vi "Autonomous Independent.vi"() -> ()   [LabVIEW 2015]
doc: "This VI is called when autonomous begins, and will automatically be terminated when autonomous ends. You can carry out timed or sensor driven robot movement independently without needing to return to the caller."
uses:
  <vilib>/Rock Robotics/WPI/Utilities/WPI_GetSetVariantRefNum.vi
  <vilib>/Rock Robotics/Network Tables/NT Write Numeric Array.vi
  <vilib>/Rock Robotics/Network Tables/NT Read String.vi
panel:
  in  "Enum 2":T1(ring)
  in  "Enum":T2(ring)
  # "Be sure to right-click and choose Data Operations>>Make Current Value default if you want to save the array values with the VI"
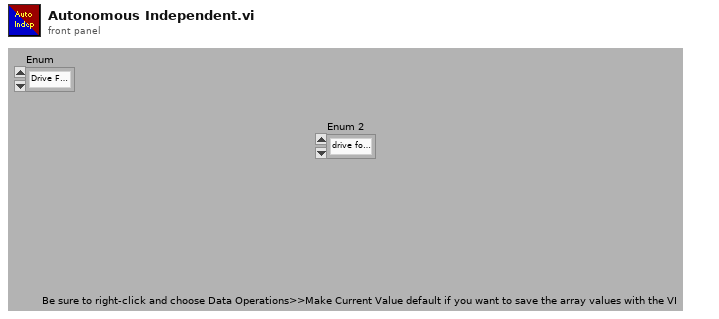
[diagram p1: front panel]
types:
  T1 = enum16{"drive forward", "extend elevator", "drive forward and hook DB", "drive backward and go down", "drive forward some"}
  T2 = enum16{"Drive Forward", "Hook Door", "Drive Backward", "Spin Longway or Something", "Drive Backwards"}
  T3 = typedef "WPI_RobotDriveDevRef.ctl" = cluster{"DevStatus":errorcluster, "Motors[]":T4[], "Square Inputs":bool, "Max Output":dbl}
  T4 = typedef "WPI_MotorControlDeviceRef.ctl" = cluster{"DeviceStatus":errorcluster, "Type":T5, "PWM":cluster{"PWM Channel":T6, "DeadBand":T7}, "CAN":cluster{"Device Number":u8, "Control Mode":T8, "Semaphore":T9, "Max Vout":dbl, "TalonSRX Control Mode":T10}, "Invert":bool}
  T5 = typedef "WPI_MotorControlType.ctl" = enum16{"PWM", "CAN", "CANTalonSRX"}
  T6 = typedef "FPGA_DIOPWMChannel.ctl" = enum8{"PWM 0", "PWM 1", "PWM 2", "PWM 3", "PWM 4", "PWM 5", "PWM 6", "PWM 7", "PWM 8", "PWM 9", "PWM MXP 0", "PWM MXP 1", "PWM MXP 2", "PWM MXP 3", "PWM MXP 4", "PWM MXP 5", "PWM MXP 6", "PWM MXP 7", "PWM MXP 8", "PWM MXP 9", "Invalid"}
  T7 = typedef "WPI_PWMDeadband.ctl" = cluster{"Name":string, "maxPositivePwm":i32, "minPositivePwm":i32, "centerPwm":i32, "maxNegativePwm":i32, "minNegativePwm":i32, "angularRange":u16}
  T8 = typedef "WPI_CANJaguar_ControlMode.ctl" = enum8{"Percent VBus", "Current", "Speed", "Position", "Voltage"}
  T9 = typedef "Semaphore RefNum" = refnum<k1>
  T10 = typedef "WPI_CANTalonSRX_APIControlMode.ctl" = enum8{"Percent VBus", "Speed", "Position", "Slave", "Unchanged / Invalid", "Voltage Compensation", "Current", "Motion Profile"}
  T11 = typedef "WPI_EncoderDevRef.ctl" = cluster{"DevStatus":errorcluster, "EncoderIndex":T12, "CounterIndex":T13, "DistancePerCount":dbl, "Decoding Type":T14}
  T12 = typedef "FPGA_EncoderIdx.ctl" = enum8{"Enc 0", "Enc 1", "Enc 2", "Enc 3", "Enc 4", "Enc 5", "Enc 6", "Enc 7", "Invalid"}
  T13 = typedef "FPGA_CounterCtrSystemIndex.ctl" = enum8{"Ctr 0", "Ctr 1", "Ctr 2", "Ctr 3", "Ctr 4", "Ctr 5", "Ctr 6", "Ctr 7", "Invalid"}
  T14 = typedef "WPI_EncoderType.ctl" = enum16{"1x", "2x", "4x"}
  T15 = typedef "WPI_JoystickDevRef.ctl" = cluster{"Device":T16}
  T16 = typedef "WPI_JoystickDeviceEnum.ctl" = enum16{"USB 0", "USB 1", "USB 2", "USB 3", "USB 4", "USB 5"}
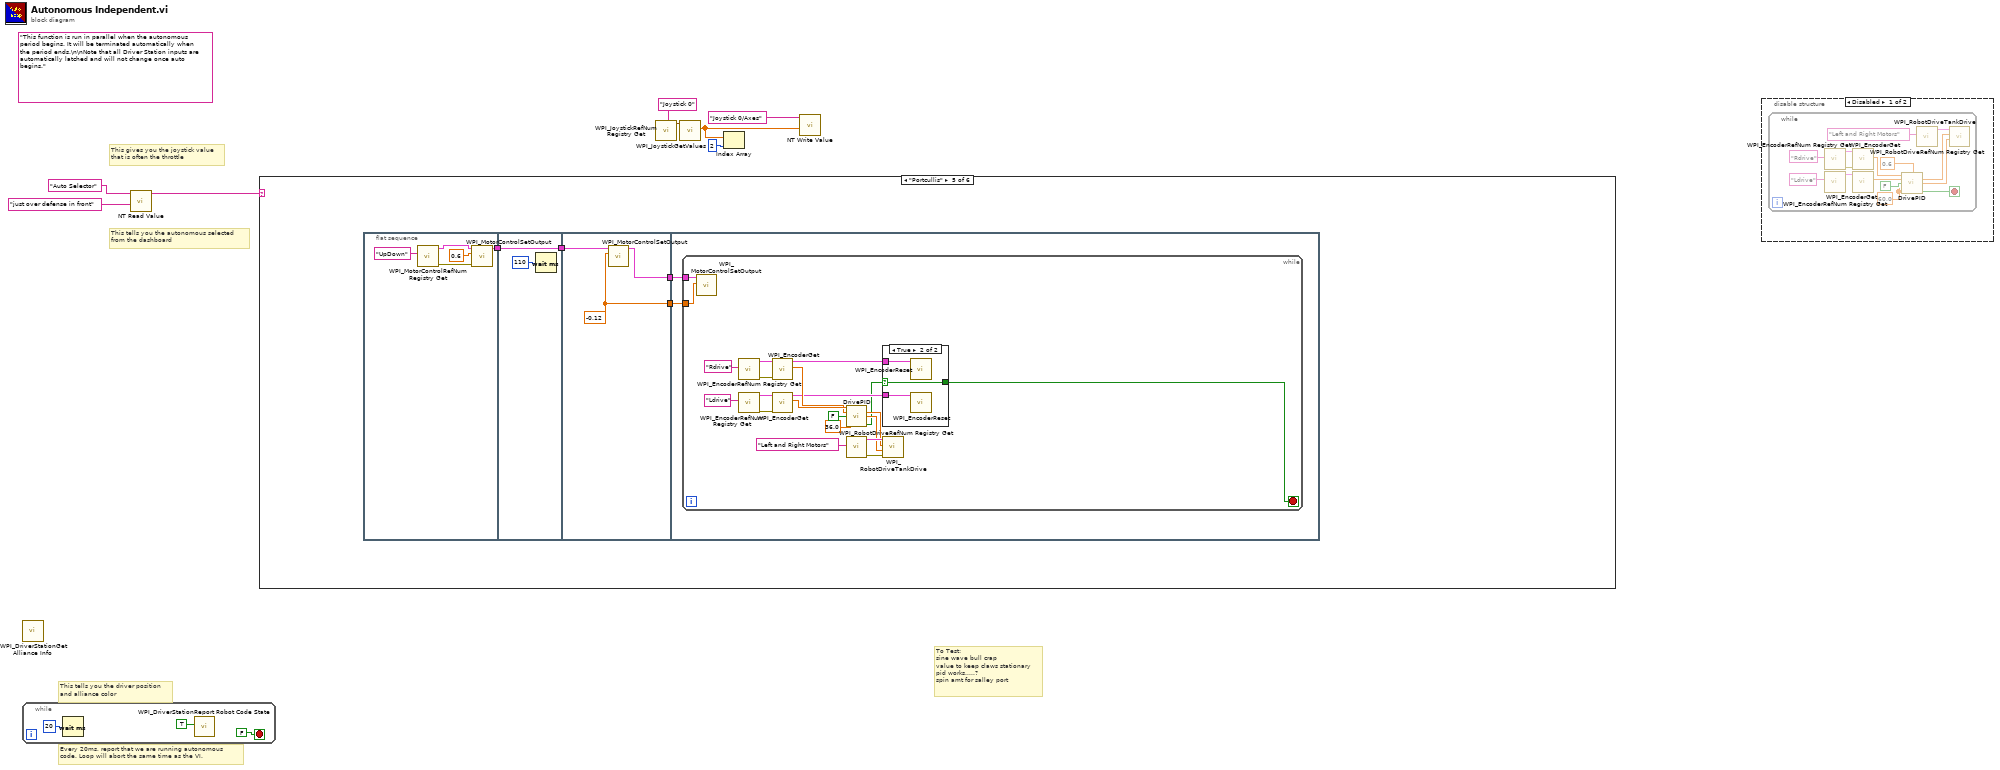
[diagram p0: block diagram]
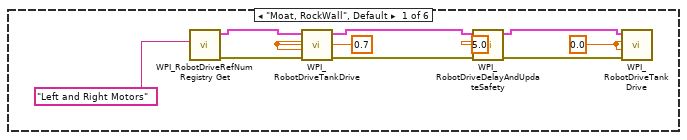
[diagram p2: hidden frame]
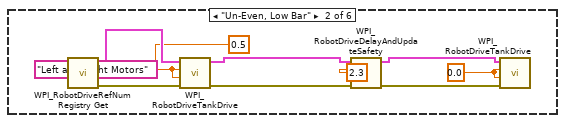
[diagram p3: hidden frame]
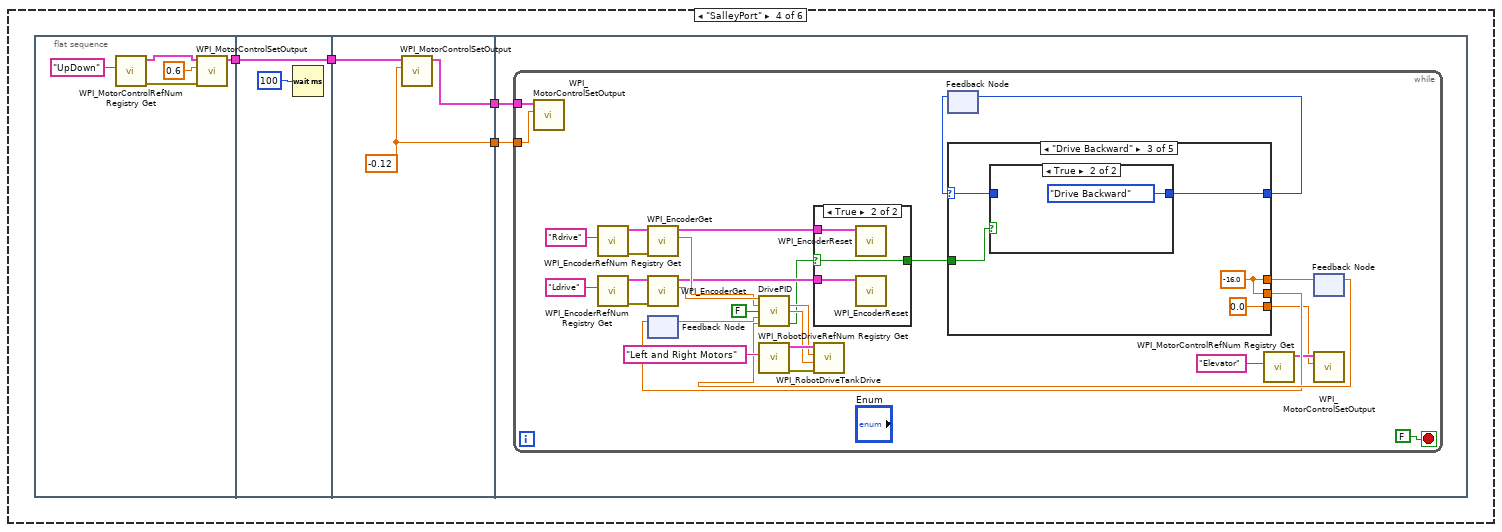
[diagram p5: hidden frame]
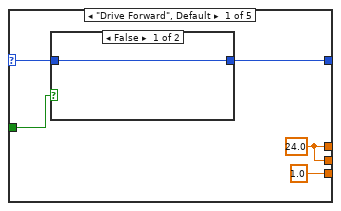
[diagram p6: hidden frame]
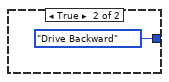
[diagram p7: hidden frame]
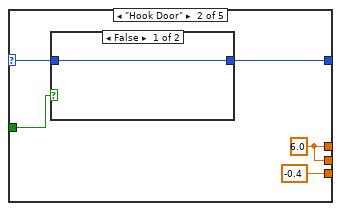
[diagram p8: hidden frame]
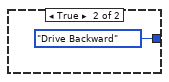
[diagram p9: hidden frame]
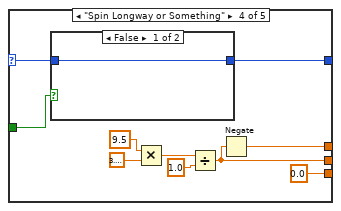
[diagram p11: hidden frame]
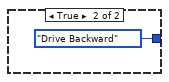
[diagram p12: hidden frame]
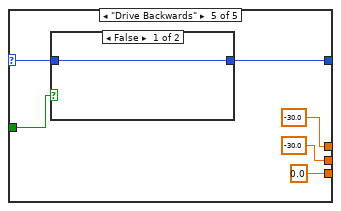
[diagram p13: hidden frame]
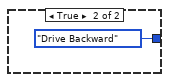
[diagram p14: hidden frame]
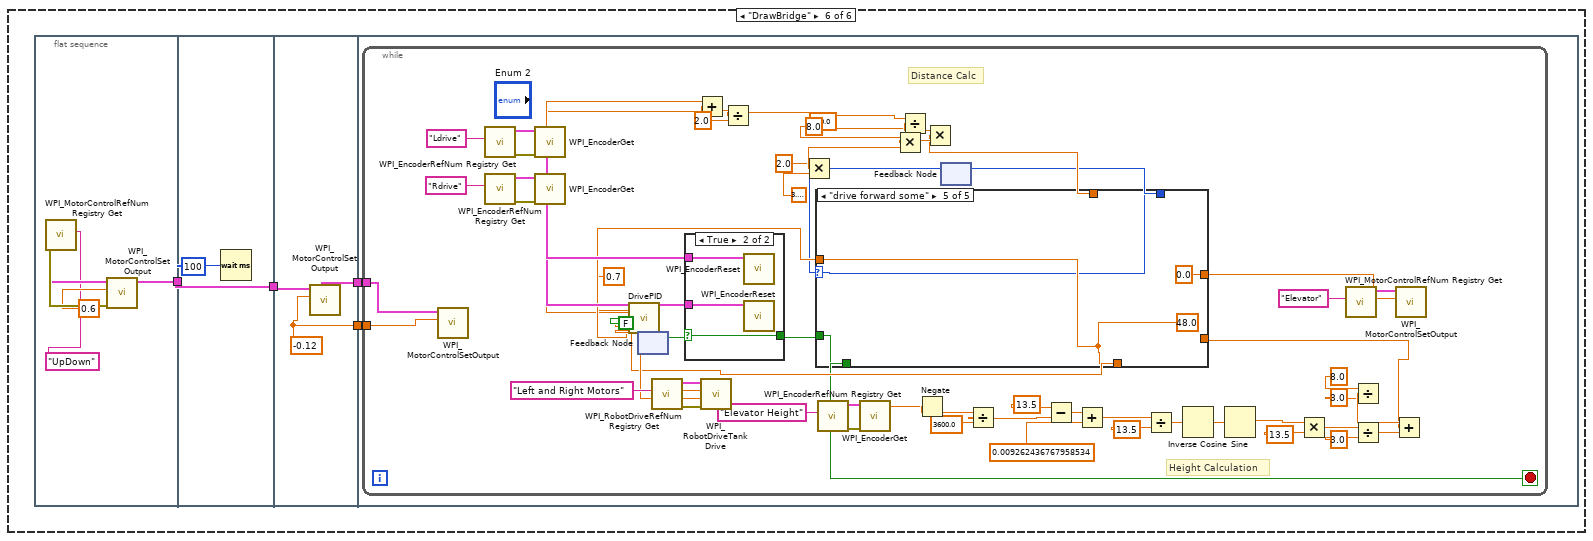
[diagram p17: hidden frame]
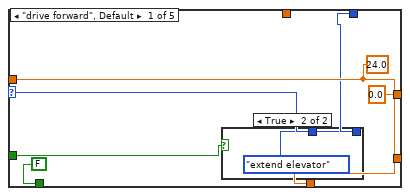
[diagram p19: hidden frame]
diagram:
  (unwired) "This function is run in parallel when the autonomous period begins. It will be terminated automatically when the period ends.\n\nNote that all Driver Station inputs are automatically latched and will not change once auto begins."
  # "To Test:\nsine wave bull crap\nvalue to keep claws stationary\npid works.....?\nspin amt for salley port"
  # "This tells you the autonomous selected\nfrom the dashboard"
  # "Every 20ms, report that we are running autonomous\ncode. Loop will abort the same time as the VI."
  # "This gives you the joystick value\nthat is often the throttle"
  # "This tells you the driver position\nand alliance color"
  n1 = while {
    stop <- FALSE stop-if-true
    n2 = Wait (ms)(milliseconds to wait=u32 20) -> ()  [unwired: 1 out]
    n3 = call <vilib>:"WPI_DriverStationReport Robot Code State.vi"("Autonomous"=TRUE) -> ()  [unwired: 10 in, 1 out]
  }
  n4 = call <vilib>:"WPI_DriverStationGet Alliance Info.vi"() -> ()  [unwired: 12 out]
  n5 = call-poly <vilib>:"NT Read Value.vi"("Default Value"="just over defense in front", "Name"="Auto Selector") -> ("String"=w1:string)  [unwired: 8 in, 1 out]
  n6 = case shown="\"Portcullis\"" w1 {
    frame "Moat, RockWall", Default {
      w15 = 0.0 ("Left axis value")
      w16 = 0.7 ("Left axis value")
      n7 = call <vilib>:"WPI_RobotDriveRefNum Registry Get.vi"("refnum name"="Left and Right Motors") -> ("error out"=w18:errorcluster, "RobotDriveDevRef"=w21:T3)  [unwired: 9 in]
      n8 = call <vilib>:"WPI_RobotDriveTankDrive.vi"("error in (no error)"=w18, "Right axis value"=w16, "Left axis value"=w16, "RobotDriveDevRef"=w21) -> ("error out"=w17:errorcluster, "RobotDriveDevRef"=w19:T3)  [unwired: 5 in, 1 out]
      n9 = call <vilib>:"WPI_RobotDriveDelayAndUpdateSafety.vi"("error in (no error)"=w17, "Delay (s)"=5.0, "RobotDriveDevRef"=w19) -> ("error out"=w13:errorcluster, "RobotDriveDevRef 2"=w14:T3)  [unwired: 7 in]
      n10 = call <vilib>:"WPI_RobotDriveTankDrive.vi"("error in (no error)"=w13, "Right axis value"=w15, "Left axis value"=w15, "RobotDriveDevRef"=w14) -> ()  [unwired: 5 in, 3 out]
    }
    frame "Un-Even, Low Bar" {
      w22 = 0.5 ("Left axis value")
      w28 = 0.0 ("Left axis value")
      n11 = call <vilib>:"WPI_RobotDriveRefNum Registry Get.vi"("refnum name"="Left and Right Motors") -> ("error out"=w26:errorcluster, "RobotDriveDevRef"=w23:T3)  [unwired: 9 in]
      n12 = call <vilib>:"WPI_RobotDriveTankDrive.vi"("error in (no error)"=w26, "Right axis value"=w22, "Left axis value"=w22, "RobotDriveDevRef"=w23) -> ("error out"=w27:errorcluster, "RobotDriveDevRef"=w25:T3)  [unwired: 5 in, 1 out]
      n13 = call <vilib>:"WPI_RobotDriveDelayAndUpdateSafety.vi"("error in (no error)"=w27, "Delay (s)"=2.3, "RobotDriveDevRef"=w25) -> ("error out"=w30:errorcluster, "RobotDriveDevRef 2"=w29:T3)  [unwired: 7 in]
      n14 = call <vilib>:"WPI_RobotDriveTankDrive.vi"("error in (no error)"=w30, "Right axis value"=w28, "Left axis value"=w28, "RobotDriveDevRef"=w29) -> ()  [unwired: 5 in, 3 out]
    }
    frame "Toaster" {
    }
    frame "SalleyPort" {
      n15 = flat-sequence {
        tunnel: [w37] -> w35
        tunnel: w35 -> [w41]
        tunnel: [w41] -> w34
        tunnel: w34 -> [w45]
        tunnel: [w44] -> w33
        tunnel: [w43] -> w32
        tunnel: w33 -> [w47]
        tunnel: w32 -> [w46]
        frame #0 {
          n16 = call <vilib>:"WPI_MotorControlRefNum Registry Get.vi"("refnum name"="UpDown") -> ("error out"=w40:errorcluster, "MotorControlDevRef"=w39:T4)  [unwired: 9 in]
          n17 = call <vilib>:"WPI_MotorControlSetOutput.vi"("error in (no error)"=w40, "Output"=0.6, "MotorControlDevRef"=w39) -> ("MotorControlDevRef"=w37:T4)  [unwired: 6 in, 2 out]
        }
        frame #1 {
          n18 = Wait (ms)(milliseconds to wait=u32 100) -> ()  [unwired: 1 out]
        }
        frame #2 {
          w43 = -0.12 ("Output")
          n19 = call <vilib>:"WPI_MotorControlSetOutput.vi"("Output"=w43, "MotorControlDevRef"=w45) -> ("MotorControlDevRef"=w44:T4)  [unwired: 7 in, 2 out]
        }
        frame #3 {
          n20 = while {
            tunnel: w47 -> [w49]
            tunnel: w46 -> [w48]
            stop <- FALSE stop-if-true
            n21 = call <vilib>:"WPI_MotorControlSetOutput.vi"("Output"=w48, "MotorControlDevRef"=w49) -> ()  [unwired: 7 in, 3 out]
            n22 = call <vilib>:"WPI_EncoderRefNum Registry Get.vi"("refnum name"="Rdrive") -> ("error out"=w74:errorcluster, "EncoderDevRef"=w73:T11)  [unwired: 9 in]
            n23 = call <vilib>:"WPI_EncoderRefNum Registry Get.vi"("refnum name"="Ldrive") -> ("error out"=w76:errorcluster, "EncoderDevRef"=w75:T11)  [unwired: 9 in]
            n24 = call <vilib>:"WPI_EncoderGet.vi"("error in (no error)"=w74, "EncoderDevRef"=w73) -> ("Distance"=w69:dbl, "EncoderDevRef"=w62:T11)  [unwired: 4 in, 4 out]
            n25 = call <vilib>:"WPI_EncoderGet.vi"("error in (no error)"=w76, "EncoderDevRef"=w75) -> ("Distance"=w70:dbl, "EncoderDevRef"=w63:T11)  [unwired: 4 in, 4 out]
            n26 = feedback #1() -> (w56:dbl)  [unwired: 1 in]
            n27 = call <vilib>:"WPI_RobotDriveRefNum Registry Get.vi"("refnum name"="Left and Right Motors") -> ("error out"=w67:errorcluster, "RobotDriveDevRef"=w66:T3)  [unwired: 9 in]
            n28 = feedback #2() -> (w54:T2)  [unwired: 1 in]
            n29 = call <vilib>:"WPI_MotorControlRefNum Registry Get.vi"("refnum name"="Elevator") -> ("MotorControlDevRef"=w52:T4)  [unwired: 9 in, 1 out]
            n30 = feedback #3() -> (w60:dbl)  [unwired: 1 in]
            n31 = call "DrivePID.vi"("Ldrive Encoder"=w70, "Rdrive Encoder"=w69, "Compensate"=FALSE, "SetpointLeft"=w56, "SetpointRight"=w60) -> ("Left Out"=w65:dbl, "Right Out"=w64:dbl, "Done"=w59:bool)  [unwired: 8 in]
            n32 = case shown="True" w59 {
              selector: w59 -> [w119 w120]
              tunnel: w63 -> [_ w122]
              tunnel: w62 -> [_ w121]
              tunnel: [w119 w120] -> w58
              frame False {
              }
              frame True {
                n33 = call <vilib>:"WPI_EncoderReset.vi"("EncoderDevRef"=w121) -> ()  [unwired: 9 in, 2 out]
                n34 = call <vilib>:"WPI_EncoderReset.vi"("EncoderDevRef"=w122) -> ()  [unwired: 9 in, 2 out]
              }
            }
            n35 = call <vilib>:"WPI_RobotDriveTankDrive.vi"("error in (no error)"=w67, "Right axis value"=w64, "Left axis value"=w65, "RobotDriveDevRef"=w66) -> ()  [unwired: 5 in, 3 out]
            n36 = case shown="\"Drive Backward\"" w54 {
              selector: w54 -> [w81 w88 w95 w107 w115]
              tunnel: [w82 w89 w96 w108 w116] -> w55
              tunnel: w58 -> [w78 w87 w94 w106 w114]
              tunnel: [w80 w85 w92 w100 -30.0] -> w61
              tunnel: [w80 w85 w92 w101 -30.0] -> w57
              tunnel: [1.0 -0.4 0.0 0.0 0.0] -> w51
              frame "Drive Forward", Default {
                w80 = 24.0
                n37 = case shown="False" w78 {
                  tunnel: [w83 T2."Drive Backward" ("Enum")] -> w82
                  tunnel: w81 -> [w83 _]
                  frame False {
                  }
                  frame True {
                  }
                }
              }
              frame "Hook Door" {
                w85 = 6.0
                n38 = case shown="False" w87 {
                  tunnel: [w90 T2."Drive Backward" ("Enum")] -> w89
                  tunnel: w88 -> [w90 _]
                  frame False {
                  }
                  frame True {
                  }
                }
              }
              frame "Drive Backward" {
                w92 = -16.0
                n39 = case shown="True" w94 {
                  tunnel: [w97 T2."Drive Backward" ("Enum")] -> w96
                  tunnel: w95 -> [w97 _]
                  frame False {
                  }
                  frame True {
                  }
                }
              }
              frame "Spin Longway or Something" {
                n40 = case shown="False" w106 {
                  tunnel: [w109 T2."Drive Backward" ("Enum")] -> w108
                  tunnel: w107 -> [w109 _]
                  frame False {
                  }
                  frame True {
                  }
                }
                n41 = Multiply(x=9.5, y=3.141592653589793) -> (x*y=w104:dbl)
                n42 = Divide(x=w104, y=1.0) -> (x/y=w101:dbl)
                n43 = Negate(x=w101) -> (-x=w100:dbl)
              }
              frame "Drive Backwards" {
                n44 = case shown="False" w114 {
                  tunnel: [w117 T2."Drive Backward" ("Enum")] -> w116
                  tunnel: w115 -> [w117 _]
                  frame False {
                  }
                  frame True {
                  }
                }
              }
            }
            n45 = feedback-in #1(w57) -> ()
            n46 = feedback-in #2(w55) -> ()
            n47 = feedback-in #3(w61) -> ()
            n48 = call <vilib>:"WPI_MotorControlSetOutput.vi"("Output"=w51, "MotorControlDevRef"=w52) -> ()  [unwired: 7 in, 3 out]
          }
        }
      }
    }
    frame "Portcullis" {
      n49 = flat-sequence {
        tunnel: [w128] -> w126
        tunnel: w126 -> [w132]
        tunnel: [w132] -> w125
        tunnel: w125 -> [w136]
        tunnel: [w135] -> w124
        tunnel: [w134] -> w123
        tunnel: w124 -> [w138]
        tunnel: w123 -> [w137]
        frame #0 {
          n50 = call <vilib>:"WPI_MotorControlRefNum Registry Get.vi"("refnum name"="UpDown") -> ("error out"=w131:errorcluster, "MotorControlDevRef"=w130:T4)  [unwired: 9 in]
          n51 = call <vilib>:"WPI_MotorControlSetOutput.vi"("error in (no error)"=w131, "Output"=0.6, "MotorControlDevRef"=w130) -> ("MotorControlDevRef"=w128:T4)  [unwired: 6 in, 2 out]
        }
        frame #1 {
          n52 = Wait (ms)(milliseconds to wait=u32 110) -> ()  [unwired: 1 out]
        }
        frame #2 {
          w134 = -0.12 ("Output")
          n53 = call <vilib>:"WPI_MotorControlSetOutput.vi"("Output"=w134, "MotorControlDevRef"=w136) -> ("MotorControlDevRef"=w135:T4)  [unwired: 7 in, 2 out]
        }
        frame #3 {
          n54 = while {
            tunnel: w138 -> [w142]
            tunnel: w137 -> [w141]
            stop <- w140 stop-if-true
            w139 = 36.0 ("SetpointLeft")
            n55 = call <vilib>:"WPI_MotorControlSetOutput.vi"("Output"=w141, "MotorControlDevRef"=w142) -> ()  [unwired: 7 in, 3 out]
            n56 = call <vilib>:"WPI_EncoderRefNum Registry Get.vi"("refnum name"="Rdrive") -> ("error out"=w156:errorcluster, "EncoderDevRef"=w155:T11)  [unwired: 9 in]
            n57 = call <vilib>:"WPI_EncoderRefNum Registry Get.vi"("refnum name"="Ldrive") -> ("error out"=w158:errorcluster, "EncoderDevRef"=w157:T11)  [unwired: 9 in]
            n58 = call <vilib>:"WPI_EncoderGet.vi"("error in (no error)"=w156, "EncoderDevRef"=w155) -> ("Distance"=w151:dbl, "EncoderDevRef"=w144:T11)  [unwired: 4 in, 4 out]
            n59 = call <vilib>:"WPI_EncoderGet.vi"("error in (no error)"=w158, "EncoderDevRef"=w157) -> ("Distance"=w152:dbl, "EncoderDevRef"=w145:T11)  [unwired: 4 in, 4 out]
            n60 = call "DrivePID.vi"("Ldrive Encoder"=w152, "Rdrive Encoder"=w151, "Compensate"=FALSE, "SetpointLeft"=w139, "SetpointRight"=w139) -> ("Left Out"=w147:dbl, "Right Out"=w146:dbl, "Done"=w143:bool)  [unwired: 8 in]
            n61 = call <vilib>:"WPI_RobotDriveRefNum Registry Get.vi"("refnum name"="Left and Right Motors") -> ("error out"=w149:errorcluster, "RobotDriveDevRef"=w148:T3)  [unwired: 9 in]
            n62 = case shown="True" w143 {
              selector: w143 -> [w160 w161]
              tunnel: w145 -> [_ w163]
              tunnel: w144 -> [_ w162]
              tunnel: [w160 w161] -> w140
              frame False {
              }
              frame True {
                n63 = call <vilib>:"WPI_EncoderReset.vi"("EncoderDevRef"=w162) -> ()  [unwired: 9 in, 2 out]
                n64 = call <vilib>:"WPI_EncoderReset.vi"("EncoderDevRef"=w163) -> ()  [unwired: 9 in, 2 out]
              }
            }
            n65 = call <vilib>:"WPI_RobotDriveTankDrive.vi"("error in (no error)"=w149, "Right axis value"=w146, "Left axis value"=w147, "RobotDriveDevRef"=w148) -> ()  [unwired: 5 in, 3 out]
          }
        }
      }
    }
    frame "DrawBridge" {
      n66 = flat-sequence {
        tunnel: [w169] -> w167
        tunnel: w167 -> [w173]
        tunnel: [w173] -> w166
        tunnel: w166 -> [w177]
        tunnel: [w176] -> w165
        tunnel: [w175] -> w164
        tunnel: w165 -> [w179]
        tunnel: w164 -> [w178]
        frame #0 {
          n67 = call <vilib>:"WPI_MotorControlRefNum Registry Get.vi"("refnum name"="UpDown") -> ("error out"=w172:errorcluster, "MotorControlDevRef"=w171:T4)  [unwired: 9 in]
          n68 = call <vilib>:"WPI_MotorControlSetOutput.vi"("error in (no error)"=w172, "Output"=0.6, "MotorControlDevRef"=w171) -> ("MotorControlDevRef"=w169:T4)  [unwired: 6 in, 2 out]
        }
        frame #1 {
          n69 = Wait (ms)(milliseconds to wait=u32 100) -> ()  [unwired: 1 out]
        }
        frame #2 {
          w175 = -0.12 ("Output")
          n70 = call <vilib>:"WPI_MotorControlSetOutput.vi"("Output"=w175, "MotorControlDevRef"=w177) -> ("MotorControlDevRef"=w176:T4)  [unwired: 7 in, 2 out]
        }
        frame #3 {
          n71 = while {
            tunnel: w179 -> [w181]
            tunnel: w178 -> [w180]
            stop <- w208 stop-if-true
            # "Height Calculation"
            # "Distance Calc"
            n72 = call <vilib>:"WPI_MotorControlSetOutput.vi"("Output"=w180, "MotorControlDevRef"=w181) -> ()  [unwired: 7 in, 3 out]
            n73 = call <vilib>:"WPI_EncoderRefNum Registry Get.vi"("refnum name"="Ldrive") -> ("error out"=w239:errorcluster, "EncoderDevRef"=w238:T11)  [unwired: 9 in]
            n74 = call <vilib>:"WPI_EncoderRefNum Registry Get.vi"("refnum name"="Rdrive") -> ("error out"=w237:errorcluster, "EncoderDevRef"=w236:T11)  [unwired: 9 in]
            n75 = call <vilib>:"WPI_EncoderGet.vi"("error in (no error)"=w239, "EncoderDevRef"=w238) -> ("Distance"=w214:dbl, "EncoderDevRef"=w228:T11)  [unwired: 4 in, 4 out]
            n76 = call <vilib>:"WPI_EncoderGet.vi"("error in (no error)"=w237, "EncoderDevRef"=w236) -> ("Distance"=w213:dbl, "EncoderDevRef"=w227:T11)  [unwired: 4 in, 4 out]
            n77 = feedback #4() -> (w206:bool)  [unwired: 1 in]
            n78 = call <vilib>:"WPI_RobotDriveRefNum Registry Get.vi"("refnum name"="Left and Right Motors") -> ("error out"=w232:errorcluster, "RobotDriveDevRef"=w231:T3)  [unwired: 9 in]
            n79 = case shown="True" w206 {
              selector: w206 -> [w244 w245]
              tunnel: w228 -> [_ w247]
              tunnel: w227 -> [_ w246]
              tunnel: [w244 w245] -> w226
              frame False {
              }
              frame True {
                n80 = call <vilib>:"WPI_EncoderReset.vi"("EncoderDevRef"=w247) -> ()  [unwired: 9 in, 2 out]
                n81 = call <vilib>:"WPI_EncoderReset.vi"("EncoderDevRef"=w246) -> ()  [unwired: 9 in, 2 out]
              }
            }
            n82 = Add(x=w214, y=w213) -> (x+y=w215:dbl)
            n83 = Divide(x=w215, y=2.0) -> (x/y=w212:dbl)
            n84 = Multiply(x=2.0, y=3.141592653589793) -> (x*y=w221:dbl)
            n85 = call <vilib>:"WPI_EncoderRefNum Registry Get.vi"("refnum name"="Elevator Height") -> ("error out"=w185:errorcluster, "EncoderDevRef"=w186:T11)  [unwired: 9 in]
            n86 = call <vilib>:"WPI_EncoderGet.vi"("error in (no error)"=w185, "EncoderDevRef"=w186) -> ("Distance"=w197:dbl)  [unwired: 4 in, 5 out]
            n87 = Multiply(x=8.0, y=w221) -> (x*y=w219:dbl)
            n88 = Divide(x=w212, y=720.0) -> (x/y=w218:dbl)
            n89 = Negate(x=w197) -> (-x=w202:dbl)
            n90 = Multiply(x=w218, y=w219) -> (x*y=w211:dbl)
            n91 = feedback #5() -> (w209:T1)  [unwired: 1 in]
            n92 = Divide(x=w202, y=3600.0 ("x")) -> (x/y=w192:dbl)
            n93 = Subtract(x=13.5, y=w192) -> (x-y=w194:dbl)
            n94 = Add(x=w194, y=0.009262436767958534) -> (x+y=w195:dbl)
            n95 = Divide(x=w195, y=13.5) -> (x/y=w188:dbl)
            n96 = Inverse Cosine(1:w188) -> (0:w189:dbl)
            n97 = Sine(x=w189) -> (sin(x)=w190:dbl)
            n98 = Multiply(x=w190, y=13.5) -> (x*y=w201:dbl)
            n99 = call <vilib>:"WPI_MotorControlRefNum Registry Get.vi"("refnum name"="Elevator") -> ("MotorControlDevRef"=w243:T4)  [unwired: 9 in, 1 out]
            n100 = Divide(x=8.0, y=3.0) -> (x/y=w205:dbl)
            n101 = Divide(x=w201, y=3.0) -> (x/y=w199:dbl)
            n102 = Add(x=w205, y=w199) -> (x+y=w183:dbl)
            n103 = case shown="\"drive forward some\"" w209 {
              selector: w209 -> [w249 w258 w269 w277 w290]
              tunnel: [0.0 ("Output") w261 0.0 ("Output") w282 0.0 ("Output")] -> w241
              tunnel: [w251 w260 w273 w281 w291] -> w224
              tunnel: [w251 w260 w273 w281 w291] -> w225
              tunnel: w226 -> [w252 _ w271 w279 w289]
              tunnel: w211 -> [_ _ _ w280 _]
              tunnel: [w250 w259 w270 w278 w290] -> w210
              tunnel: [FALSE FALSE FALSE FALSE w289] -> w208
              tunnel: w183 -> [_ w256 _ _ _]
              frame "drive forward", Default {
                w251 = 24.0
                n104 = case shown="True" w252 {
                  tunnel: [w254 T1."extend elevator" ("Enum 2")] -> w250
                  tunnel: w249 -> [w254 _]
                  frame False {
                  }
                  frame True {
                  }
                }
              }
              frame "extend elevator" {
                w260 = 0.0
                n105 = Less?(x=w256, y=40.0) -> (x < y?=w262:bool)
                n106 = case shown="True" w262 {
                  tunnel: [1.0 ("Output") 0.0 ("Output")] -> w261
                  tunnel: [w264 T1."drive forward and hook DB" ("Enum 2")] -> w259
                  tunnel: w258 -> [w264 _]
                  frame False {
                  }
                  frame True {
                  }
                }
              }
              frame "drive forward and hook DB" {
                w273 = 12.0
                n107 = case shown="True" w271 {
                  tunnel: [w274 T1."drive backward and go down" ("Enum 2")] -> w270
                  tunnel: w269 -> [w274 _]
                  frame False {
                  }
                  frame True {
                  }
                }
              }
              frame "drive backward and go down" {
                w281 = -36.0
                n108 = case shown="True" w279 {
                  tunnel: [w287 T1."drive forward some" ("Enum 2")] -> w278
                  tunnel: w277 -> [w287 _]
                  frame False {
                  }
                  frame True {
                  }
                }
                n109 = Divide(x=3.141592653589793, y=72.0) -> (x/y=w285:dbl)
                n110 = Multiply(x=w285, y=w280) -> (x*y=w286:dbl)
                n111 = Sine(x=w286) -> (sin(x)=w282:dbl)
              }
              frame "drive forward some" {
                w291 = 48.0
              }
            }
            n112 = call "DrivePID.vi"("Ldrive Encoder"=w214, "Max Speed"=0.7, "Rdrive Encoder"=w213, "Compensate"=FALSE, "SetpointLeft"=w224, "SetpointRight"=w225) -> ("Left Out"=w230:dbl, "Right Out"=w229:dbl, "Done"=w207:bool)  [unwired: 7 in]
            n113 = feedback-in #4(w207) -> ()
            n114 = call <vilib>:"WPI_RobotDriveTankDrive.vi"("error in (no error)"=w232, "Right axis value"=w229, "Left axis value"=w230, "RobotDriveDevRef"=w231) -> ()  [unwired: 5 in, 3 out]
            n115 = feedback-in #5(w210) -> ()
            n116 = call <vilib>:"WPI_MotorControlSetOutput.vi"("Output"=w241, "MotorControlDevRef"=w243) -> ()  [unwired: 7 in, 3 out]
          }
        }
      }
    }
  }
  n117 = call <vilib>:"WPI_JoystickRefNum Registry Get.vi"("refnum name"="Joystick 0") -> ("JoystickDevRef"=w7:T15)  [unwired: 1 in, 9 out]
  n118 = call <vilib>:"WPI_JoystickGetValues.vi"("JoystickDevRef"=w7) -> ("Axes"=w5:dbl[])  [unwired: 6 in, 4 out]
  n119 = Index Array(array=w5, index=2) -> ()  [unwired: 1 out]
  n120 = call-poly <vilib>:"NT Write Value.vi"("Numeric Array"=w5, "Name"="Joystick 0/Axes") -> ()  [unwired: 9 in, 1 out]
  n121 = disable-structure shown="Disabled" {
    frame Disabled {
      n122 = while {
        stop <- w306 stop-if-true
        w305 = 60.0 ("SetpointLeft")
        n123 = call <vilib>:"WPI_EncoderRefNum Registry Get.vi"("refnum name"="Rdrive") -> ("error out"=w300:errorcluster, "EncoderDevRef"=w299:T11)  [unwired: 9 in]
        n124 = call <vilib>:"WPI_EncoderRefNum Registry Get.vi"("refnum name"="Ldrive") -> ("EncoderDevRef"=w298:T11)  [unwired: 9 in, 1 out]
        n125 = call <vilib>:"WPI_EncoderGet.vi"("error in (no error)"=w300, "EncoderDevRef"=w299) -> ("Distance"=w295:dbl)  [unwired: 4 in, 5 out]
        n126 = call <vilib>:"WPI_EncoderGet.vi"("EncoderDevRef"=w298) -> ("Distance"=w296:dbl)  [unwired: 5 in, 5 out]
        n127 = call "DrivePID.vi"("Ldrive Encoder"=w295, "Max Speed"=0.6, "Rdrive Encoder"=w296, "Compensate"=FALSE, "SetpointLeft"=w305, "SetpointRight"=w305) -> ("Left Out"=w302:dbl, "Right Out"=w301:dbl, "Done"=w306:bool)  [unwired: 7 in]
        n128 = call <vilib>:"WPI_RobotDriveRefNum Registry Get.vi"("refnum name"="Left and Right Motors") -> ("RobotDriveDevRef"=w303:T3)  [unwired: 1 in, 9 out]
        n129 = call <vilib>:"WPI_RobotDriveTankDrive.vi"("Right axis value"=w301, "Left axis value"=w302, "RobotDriveDevRef"=w303) -> ()  [unwired: 6 in, 3 out]
      }
    }
    frame Enabled {
    }
  }
